vi "BuildHexString.vi"(11 "Binary":string) -> (3 "String":string)   [LabVIEW 2019]
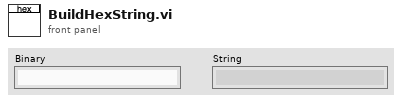
[diagram p1: front panel]
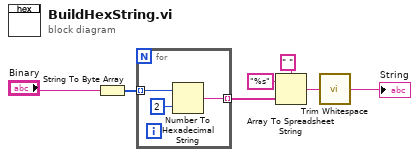
[diagram p0: block diagram]
diagram:
  n1 = String To Byte Array(string="Binary") -> (unsigned byte array=w6:u8[])
  n2 = for {
    tunnel: [w10] -> w5 mode=indexing
    tunnel: w6 -> [w9] mode=indexing
    n3 = Number To Hexadecimal String(1:i16 2 ("width (-)"), 2:w9) -> (0:w10:string)
  }
  n4 = Array To Spreadsheet String(delimiter (Tab)=" ", array=w5, 3:"%s" ("format string")) -> (spreadsheet string=w2:string)
  n5 = call <vilib>:"Trim Whitespace.vi"("string"=w2) -> ("trimmed string"=→"String":string)  [unwired: 1 in]
